vi "FindCameras.vi"(8 "error in (no error)":errorcluster, 10 "Address (Broadcast)":string="255.255.255.255", 11 "reference in":refnum<class "Camera_IMAQdx.lvclass">) -> (0 "error out":errorcluster, 2 "Camera Information Array":T1(array[cluster]), 3 "reference out":refnum<class "Camera_IMAQdx.lvclass">)   [LabVIEW 2017, in "Camera_IMAQdx.lvclass"]
doc: "Finds any ethernet cameras connected to the computer network"
uses:
  Camera_IMAQdx.lvclass
  <vilib>/vision/driver/NI_Vision_Acquisition_Software.lvlib
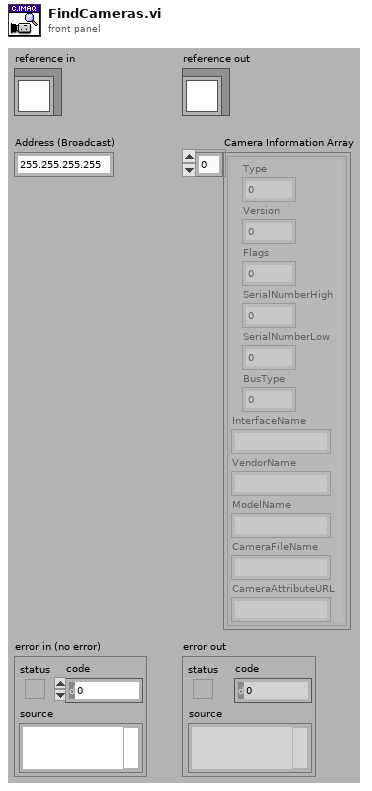
[diagram p1: front panel]
types:
  T1 = cluster{"Type":u32, "Version":u32, "Flags":u32, "SerialNumberHigh":u32, "SerialNumberLow":u32, "BusType":u32, "InterfaceName":string, "VendorName":string, "ModelName":string, "CameraFileName":string, "CameraAttributeURL":string}[]
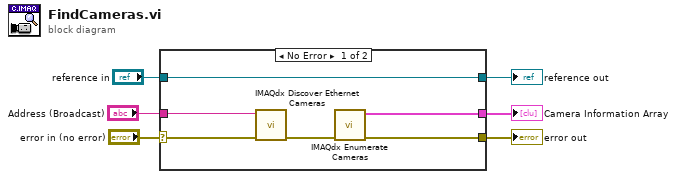
[diagram p0: block diagram]
diagram:
  n1 = case shown="No Error" "error in (no error)" {
    selector: "error in (no error)" -> [w11 w14]
    tunnel: [w9 w14] -> w5
    tunnel: [w12 w13] -> w3
    tunnel: "reference in" -> [w12 w13]
    tunnel: "Address (Broadcast)" -> [w8 _]
    tunnel: [w7 _] -> w1
    frame No Error {
      n2 = call <vilib>:"IMAQdx Discover Ethernet Cameras.vi"("error in"=w11, "Address (Broadcast)"=w8) -> ("error out"=w10:errorcluster)  [unwired: 9 in]
      n3 = call <vilib>:"IMAQdx Enumerate Cameras.vi"("error in"=w10) -> ("error out"=w9:errorcluster, "Camera Information Array"=w7:T1)  [unwired: 9 in]
    }
    frame Error {
    }
  }
  "error out" <- w5
  "reference out" <- w3
  "Camera Information Array" <- w1
